vi "Check Variant Data.vi"(3 "Variant Data":variant, 5 "Dataset":T2) -> (0 "Element Type":T1, 1 "Valid Type?":bool, 2 "Number of Dimensions":i32)   [LabVIEW 2018, in "vis3d.lvlib" / "CubeLogger.lvclass"]
uses:
  CubeLogger.lvclass
  Dataset.ctl
  <vilib>/Utility/Data Type/Type Definitions/Data Type.ctl
  <vilib>/Utility/Data Type/NI_Data Type.lvlib
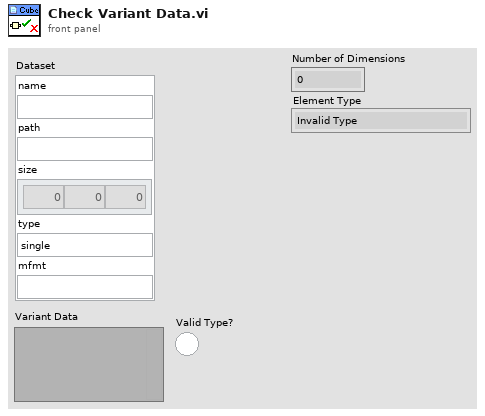
[diagram p1: front panel]
types:
  T1 = typedef "NI_Data Type.lvlib/Data Type.ctl" = enum8{"Invalid Type", "Void", "I8", "I16", "I32", "I64", "U8", "U16", "U32", "U64", "Single Float", "Double Float", "Extended Float", "Single Complex", "Double Complex", "Extended Complex", "Enum U8", "Enum U16", "Enum U32", "Enum U64", "Single Float With Unit", "Double Float With Unit", "Extended Float With Unit", "Single Complex with Unit", "Double Complex with Unit", "Extended Complex with Unit", "Boolean", "String", "Path", "Picture", "Tag", "Array", "Cluster", "Variant", "LV Variant", "Waveform", "Timestamp", "Digital Waveform", "Digital Data", "ExpressData", "Refnum", "External Data", "VI", "Poly VI", "LabVIEW Class Instance", "Fixed Point"}
  T2 = typedef "vis3d.lvlib/CubeLogger.lvclass/Dataset.ctl" = cluster{"name":string, "path":string, "size":i32[], "type":enum16{"single", "double", "uint8", "uint16", "uint32", "uint64", "int8", "int16", "int32", "int64"}, "mfmt":string}
  T3 = enum16{"single", "double", "uint8", "uint16", "uint32", "uint64", "int8", "int16", "int32", "int64"}
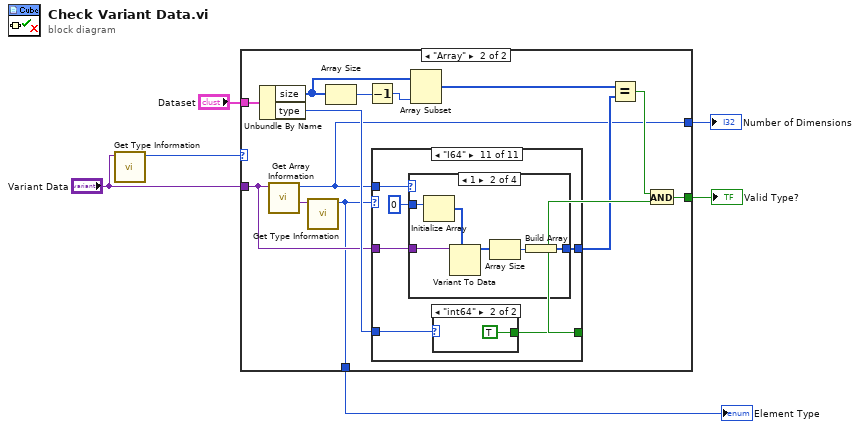
[diagram p0: block diagram]
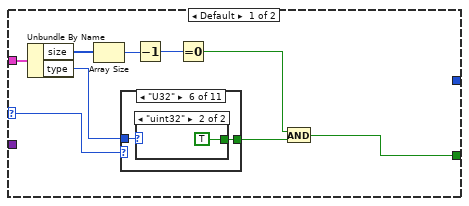
[diagram p2: hidden frame]
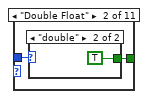
[diagram p4: hidden frame]
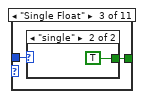
[diagram p6: hidden frame]
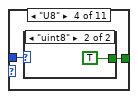
[diagram p8: hidden frame]
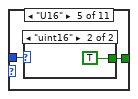
[diagram p10: hidden frame]
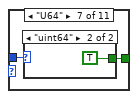
[diagram p13: hidden frame]
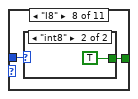
[diagram p15: hidden frame]
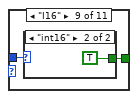
[diagram p17: hidden frame]
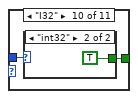
[diagram p19: hidden frame]
diagram:
  n1 = call <vilib>:"Get Type Information.vi"("Variant"="Variant Data") -> ("Type"=w6:T1)  [unwired: 6 in, 4 out]
  n2 = case shown="\"Array\"" w6 {
    selector: w6 -> [w13 _]
    tunnel: [w8 w57] -> w3
    tunnel: "Variant Data" -> [_ w49]
    tunnel: "Dataset" -> [w15 w59]
    tunnel: [_ w47] -> w2
    tunnel: [_ w46] -> w1
    frame Default {
      n3 = Unbundle By Name(w15) -> ("size"=w12:i32[], "type"=w14:T3)
      n4 = Array Size(array=w12) -> (size(s)=w11:i32)
      n5 = case shown="\"U32\"" w13 {
        tunnel: [_ w16 w19 w22 w25 w28 w31 w34 w37 w40 w43] -> w9
        tunnel: w14 -> [_ w17 w20 w23 w26 w29 w32 w35 w38 w41 w44]
        frame "Invalid Type", Default {
        }
        frame "Double Float" {
          n6 = case shown="\"double\"" w17 {
            tunnel: [_ TRUE] -> w16
            frame Default {
            }
            frame "double" {
            }
          }
        }
        frame "Single Float" {
          n7 = case shown="\"single\"" w20 {
            tunnel: [_ TRUE] -> w19
            frame Default {
            }
            frame "single" {
            }
          }
        }
        frame "U8" {
          n8 = case shown="\"uint8\"" w23 {
            tunnel: [_ TRUE] -> w22
            frame Default {
            }
            frame "uint8" {
            }
          }
        }
        frame "U16" {
          n9 = case shown="\"uint16\"" w26 {
            tunnel: [_ TRUE] -> w25
            frame Default {
            }
            frame "uint16" {
            }
          }
        }
        frame "U32" {
          n10 = case shown="\"uint32\"" w29 {
            tunnel: [_ TRUE] -> w28
            frame Default {
            }
            frame "uint32" {
            }
          }
        }
        frame "U64" {
          n11 = case shown="\"uint64\"" w32 {
            tunnel: [_ TRUE] -> w31
            frame Default {
            }
            frame "uint64" {
            }
          }
        }
        frame "I8" {
          n12 = case shown="\"int8\"" w35 {
            tunnel: [_ TRUE] -> w34
            frame Default {
            }
            frame "int8" {
            }
          }
        }
        frame "I16" {
          n13 = case shown="\"int16\"" w38 {
            tunnel: [_ TRUE] -> w37
            frame Default {
            }
            frame "int16" {
            }
          }
        }
        frame "I32" {
          n14 = case shown="\"int32\"" w41 {
            tunnel: [_ TRUE] -> w40
            frame Default {
            }
            frame "int32" {
            }
          }
        }
        frame "I64" {
          n15 = case shown="\"int64\"" w44 {
            tunnel: [_ TRUE] -> w43
            frame Default {
            }
            frame "int64" {
            }
          }
        }
      }
      n16 = Decrement(x=w11) -> (x-1=w10:i32)
      n17 = Equal To 0?(x=w10) -> (x = 0?=w7:bool)
      n18 = And(x=w7, y=w9) -> (x .and. y?=w8:bool)
    }
    frame "Array" {
      n19 = Unbundle By Name(w59) -> ("size"=w52:i32[], "type"=w54:T3)
      n20 = call <vilib>:"Get Array Information.vi"("Variant"=w49) -> ("Array Element Data Type"=w56:variant, "Number of Dimensions"=w47:i32)  [unwired: 7 in, 2 out]
      n21 = call <vilib>:"Get Type Information.vi"("Variant"=w56) -> ("Type"=w46:T1)  [unwired: 6 in, 4 out]
      n22 = Array Size(array=w52) -> (size(s)=w50:i32)
      n23 = Decrement(x=w50) -> (x-1=w51:i32)
      n24 = case shown="\"I64\"" w46 {
        tunnel: [_ w64 w87 w110 w133 w156 w179 w202 w225 w248 w271] -> w55
        tunnel: w54 -> [_ w65 w88 w111 w134 w157 w180 w203 w226 w249 w272]
        tunnel: w47 -> [_ w63 w86 w109 w132 w155 w178 w201 w224 w247 w270]
        tunnel: w49 -> [_ w61 w84 w107 w130 w153 w176 w199 w222 w245 w268]
        tunnel: [_ w60 w83 w106 w129 w152 w175 w198 w221 w244 w267] -> w48
        frame "Invalid Type", Default {
        }
        frame "Double Float" {
          n25 = case shown="1" w63 {
            tunnel: 0.0 -> [_ w69 w74 w79]
            tunnel: [_ w66 w72 w77] -> w60
            tunnel: w61 -> [_ w67 w73 w78]
            frame Default {
            }
            frame 1 {
              n26 = Initialize Array(w69) -> (w71:dbl[])  [unwired: 1 in]
              n27 = Variant To Data(type=w71, Variant=w67) -> (data=w70:dbl[])  [unwired: 1 in, 1 out]
              n28 = Array Size(array=w70) -> (size(s)=w68:i32)
              n29 = Build Array(w68) -> (w66:i32[])
            }
            frame 2 {
              n30 = Initialize Array(w74) -> (w76:dbl[][])  [unwired: 2 in]
              n31 = Variant To Data(type=w76, Variant=w73) -> (data=w75:dbl[][])  [unwired: 1 in, 1 out]
              n32 = Array Size(array=w75) -> (size(s)=w72:i32[])
            }
            frame 3 {
              n33 = Initialize Array(w79) -> (w81:dbl[][][])  [unwired: 3 in]
              n34 = Variant To Data(type=w81, Variant=w78) -> (data=w80:dbl[][][])  [unwired: 1 in, 1 out]
              n35 = Array Size(array=w80) -> (size(s)=w77:i32[])
            }
          }
          n36 = case shown="\"double\"" w65 {
            tunnel: [_ TRUE] -> w64
            frame Default {
            }
            frame "double" {
            }
          }
        }
        frame "Single Float" {
          n37 = case shown="1" w86 {
            tunnel: sgl 0.0 -> [_ w92 w97 w102]
            tunnel: [_ w89 w95 w100] -> w83
            tunnel: w84 -> [_ w90 w96 w101]
            frame Default {
            }
            frame 1 {
              n38 = Initialize Array(w92) -> (w94:sgl[])  [unwired: 1 in]
              n39 = Variant To Data(type=w94, Variant=w90) -> (data=w93:sgl[])  [unwired: 1 in, 1 out]
              n40 = Array Size(array=w93) -> (size(s)=w91:i32)
              n41 = Build Array(w91) -> (w89:i32[])
            }
            frame 2 {
              n42 = Initialize Array(w97) -> (w99:sgl[][])  [unwired: 2 in]
              n43 = Variant To Data(type=w99, Variant=w96) -> (data=w98:sgl[][])  [unwired: 1 in, 1 out]
              n44 = Array Size(array=w98) -> (size(s)=w95:i32[])
            }
            frame 3 {
              n45 = Initialize Array(w102) -> (w104:sgl[][][])  [unwired: 3 in]
              n46 = Variant To Data(type=w104, Variant=w101) -> (data=w103:sgl[][][])  [unwired: 1 in, 1 out]
              n47 = Array Size(array=w103) -> (size(s)=w100:i32[])
            }
          }
          n48 = case shown="\"single\"" w88 {
            tunnel: [_ TRUE] -> w87
            frame Default {
            }
            frame "single" {
            }
          }
        }
        frame "U8" {
          n49 = case shown="1" w109 {
            tunnel: u8 0 -> [_ w115 w120 w125]
            tunnel: [_ w112 w118 w123] -> w106
            tunnel: w107 -> [_ w113 w119 w124]
            frame Default {
            }
            frame 1 {
              n50 = Initialize Array(w115) -> (w117:u8[])  [unwired: 1 in]
              n51 = Variant To Data(type=w117, Variant=w113) -> (data=w116:u8[])  [unwired: 1 in, 1 out]
              n52 = Array Size(array=w116) -> (size(s)=w114:i32)
              n53 = Build Array(w114) -> (w112:i32[])
            }
            frame 2 {
              n54 = Initialize Array(w120) -> (w122:u8[][])  [unwired: 2 in]
              n55 = Variant To Data(type=w122, Variant=w119) -> (data=w121:u8[][])  [unwired: 1 in, 1 out]
              n56 = Array Size(array=w121) -> (size(s)=w118:i32[])
            }
            frame 3 {
              n57 = Initialize Array(w125) -> (w127:u8[][][])  [unwired: 3 in]
              n58 = Variant To Data(type=w127, Variant=w124) -> (data=w126:u8[][][])  [unwired: 1 in, 1 out]
              n59 = Array Size(array=w126) -> (size(s)=w123:i32[])
            }
          }
          n60 = case shown="\"uint8\"" w111 {
            tunnel: [_ TRUE] -> w110
            frame Default {
            }
            frame "uint8" {
            }
          }
        }
        frame "U16" {
          n61 = case shown="1" w132 {
            tunnel: u16 0 -> [_ w138 w143 w148]
            tunnel: [_ w135 w141 w146] -> w129
            tunnel: w130 -> [_ w136 w142 w147]
            frame Default {
            }
            frame 1 {
              n62 = Initialize Array(w138) -> (w140:u16[])  [unwired: 1 in]
              n63 = Variant To Data(type=w140, Variant=w136) -> (data=w139:u16[])  [unwired: 1 in, 1 out]
              n64 = Array Size(array=w139) -> (size(s)=w137:i32)
              n65 = Build Array(w137) -> (w135:i32[])
            }
            frame 2 {
              n66 = Initialize Array(w143) -> (w145:u16[][])  [unwired: 2 in]
              n67 = Variant To Data(type=w145, Variant=w142) -> (data=w144:u16[][])  [unwired: 1 in, 1 out]
              n68 = Array Size(array=w144) -> (size(s)=w141:i32[])
            }
            frame 3 {
              n69 = Initialize Array(w148) -> (w150:u16[][][])  [unwired: 3 in]
              n70 = Variant To Data(type=w150, Variant=w147) -> (data=w149:u16[][][])  [unwired: 1 in, 1 out]
              n71 = Array Size(array=w149) -> (size(s)=w146:i32[])
            }
          }
          n72 = case shown="\"uint16\"" w134 {
            tunnel: [_ TRUE] -> w133
            frame Default {
            }
            frame "uint16" {
            }
          }
        }
        frame "U32" {
          n73 = case shown="1" w155 {
            tunnel: u32 0 -> [_ w161 w166 w171]
            tunnel: [_ w158 w164 w169] -> w152
            tunnel: w153 -> [_ w159 w165 w170]
            frame Default {
            }
            frame 1 {
              n74 = Initialize Array(w161) -> (w163:u32[])  [unwired: 1 in]
              n75 = Variant To Data(type=w163, Variant=w159) -> (data=w162:u32[])  [unwired: 1 in, 1 out]
              n76 = Array Size(array=w162) -> (size(s)=w160:i32)
              n77 = Build Array(w160) -> (w158:i32[])
            }
            frame 2 {
              n78 = Initialize Array(w166) -> (w168:u32[][])  [unwired: 2 in]
              n79 = Variant To Data(type=w168, Variant=w165) -> (data=w167:u32[][])  [unwired: 1 in, 1 out]
              n80 = Array Size(array=w167) -> (size(s)=w164:i32[])
            }
            frame 3 {
              n81 = Initialize Array(w171) -> (w173:u32[][][])  [unwired: 3 in]
              n82 = Variant To Data(type=w173, Variant=w170) -> (data=w172:u32[][][])  [unwired: 1 in, 1 out]
              n83 = Array Size(array=w172) -> (size(s)=w169:i32[])
            }
          }
          n84 = case shown="\"uint32\"" w157 {
            tunnel: [_ TRUE] -> w156
            frame Default {
            }
            frame "uint32" {
            }
          }
        }
        frame "U64" {
          n85 = case shown="1" w178 {
            tunnel: u64 0 -> [_ w184 w189 w194]
            tunnel: [_ w181 w187 w192] -> w175
            tunnel: w176 -> [_ w182 w188 w193]
            frame Default {
            }
            frame 1 {
              n86 = Initialize Array(w184) -> (w186:u64[])  [unwired: 1 in]
              n87 = Variant To Data(type=w186, Variant=w182) -> (data=w185:u64[])  [unwired: 1 in, 1 out]
              n88 = Array Size(array=w185) -> (size(s)=w183:i32)
              n89 = Build Array(w183) -> (w181:i32[])
            }
            frame 2 {
              n90 = Initialize Array(w189) -> (w191:u64[][])  [unwired: 2 in]
              n91 = Variant To Data(type=w191, Variant=w188) -> (data=w190:u64[][])  [unwired: 1 in, 1 out]
              n92 = Array Size(array=w190) -> (size(s)=w187:i32[])
            }
            frame 3 {
              n93 = Initialize Array(w194) -> (w196:u64[][][])  [unwired: 3 in]
              n94 = Variant To Data(type=w196, Variant=w193) -> (data=w195:u64[][][])  [unwired: 1 in, 1 out]
              n95 = Array Size(array=w195) -> (size(s)=w192:i32[])
            }
          }
          n96 = case shown="\"uint64\"" w180 {
            tunnel: [_ TRUE] -> w179
            frame Default {
            }
            frame "uint64" {
            }
          }
        }
        frame "I8" {
          n97 = case shown="1" w201 {
            tunnel: i8 0 -> [_ w207 w212 w217]
            tunnel: [_ w204 w210 w215] -> w198
            tunnel: w199 -> [_ w205 w211 w216]
            frame Default {
            }
            frame 1 {
              n98 = Initialize Array(w207) -> (w209:i8[])  [unwired: 1 in]
              n99 = Variant To Data(type=w209, Variant=w205) -> (data=w208:i8[])  [unwired: 1 in, 1 out]
              n100 = Array Size(array=w208) -> (size(s)=w206:i32)
              n101 = Build Array(w206) -> (w204:i32[])
            }
            frame 2 {
              n102 = Initialize Array(w212) -> (w214:i8[][])  [unwired: 2 in]
              n103 = Variant To Data(type=w214, Variant=w211) -> (data=w213:i8[][])  [unwired: 1 in, 1 out]
              n104 = Array Size(array=w213) -> (size(s)=w210:i32[])
            }
            frame 3 {
              n105 = Initialize Array(w217) -> (w219:i8[][][])  [unwired: 3 in]
              n106 = Variant To Data(type=w219, Variant=w216) -> (data=w218:i8[][][])  [unwired: 1 in, 1 out]
              n107 = Array Size(array=w218) -> (size(s)=w215:i32[])
            }
          }
          n108 = case shown="\"int8\"" w203 {
            tunnel: [_ TRUE] -> w202
            frame Default {
            }
            frame "int8" {
            }
          }
        }
        frame "I16" {
          n109 = case shown="1" w224 {
            tunnel: i16 0 -> [_ w230 w235 w240]
            tunnel: [_ w227 w233 w238] -> w221
            tunnel: w222 -> [_ w228 w234 w239]
            frame Default {
            }
            frame 1 {
              n110 = Initialize Array(w230) -> (w232:i16[])  [unwired: 1 in]
              n111 = Variant To Data(type=w232, Variant=w228) -> (data=w231:i16[])  [unwired: 1 in, 1 out]
              n112 = Array Size(array=w231) -> (size(s)=w229:i32)
              n113 = Build Array(w229) -> (w227:i32[])
            }
            frame 2 {
              n114 = Initialize Array(w235) -> (w237:i16[][])  [unwired: 2 in]
              n115 = Variant To Data(type=w237, Variant=w234) -> (data=w236:i16[][])  [unwired: 1 in, 1 out]
              n116 = Array Size(array=w236) -> (size(s)=w233:i32[])
            }
            frame 3 {
              n117 = Initialize Array(w240) -> (w242:i16[][][])  [unwired: 3 in]
              n118 = Variant To Data(type=w242, Variant=w239) -> (data=w241:i16[][][])  [unwired: 1 in, 1 out]
              n119 = Array Size(array=w241) -> (size(s)=w238:i32[])
            }
          }
          n120 = case shown="\"int16\"" w226 {
            tunnel: [_ TRUE] -> w225
            frame Default {
            }
            frame "int16" {
            }
          }
        }
        frame "I32" {
          n121 = case shown="1" w247 {
            tunnel: 0 -> [_ w253 w258 w263]
            tunnel: [_ w250 w256 w261] -> w244
            tunnel: w245 -> [_ w251 w257 w262]
            frame Default {
            }
            frame 1 {
              n122 = Initialize Array(w253) -> (w255:i32[])  [unwired: 1 in]
              n123 = Variant To Data(type=w255, Variant=w251) -> (data=w254:i32[])  [unwired: 1 in, 1 out]
              n124 = Array Size(array=w254) -> (size(s)=w252:i32)
              n125 = Build Array(w252) -> (w250:i32[])
            }
            frame 2 {
              n126 = Initialize Array(w258) -> (w260:i32[][])  [unwired: 2 in]
              n127 = Variant To Data(type=w260, Variant=w257) -> (data=w259:i32[][])  [unwired: 1 in, 1 out]
              n128 = Array Size(array=w259) -> (size(s)=w256:i32[])
            }
            frame 3 {
              n129 = Initialize Array(w263) -> (w265:i32[][][])  [unwired: 3 in]
              n130 = Variant To Data(type=w265, Variant=w262) -> (data=w264:i32[][][])  [unwired: 1 in, 1 out]
              n131 = Array Size(array=w264) -> (size(s)=w261:i32[])
            }
          }
          n132 = case shown="\"int32\"" w249 {
            tunnel: [_ TRUE] -> w248
            frame Default {
            }
            frame "int32" {
            }
          }
        }
        frame "I64" {
          n133 = case shown="1" w270 {
            tunnel: i64 0 -> [_ w276 w281 w286]
            tunnel: [_ w273 w279 w284] -> w267
            tunnel: w268 -> [_ w274 w280 w285]
            frame Default {
            }
            frame 1 {
              n134 = Initialize Array(w276) -> (w278:i64[])  [unwired: 1 in]
              n135 = Variant To Data(type=w278, Variant=w274) -> (data=w277:i64[])  [unwired: 1 in, 1 out]
              n136 = Array Size(array=w277) -> (size(s)=w275:i32)
              n137 = Build Array(w275) -> (w273:i32[])
            }
            frame 2 {
              n138 = Initialize Array(w281) -> (w283:i64[][])  [unwired: 2 in]
              n139 = Variant To Data(type=w283, Variant=w280) -> (data=w282:i64[][])  [unwired: 1 in, 1 out]
              n140 = Array Size(array=w282) -> (size(s)=w279:i32[])
            }
            frame 3 {
              n141 = Initialize Array(w286) -> (w288:i64[][][])  [unwired: 3 in]
              n142 = Variant To Data(type=w288, Variant=w285) -> (data=w287:i64[][][])  [unwired: 1 in, 1 out]
              n143 = Array Size(array=w287) -> (size(s)=w284:i32[])
            }
          }
          n144 = case shown="\"int64\"" w272 {
            tunnel: [_ TRUE] -> w271
            frame Default {
            }
            frame "int64" {
            }
          }
        }
      }
      n145 = Array Subset(array=w52, length=w51) -> (w53:i32[])  [unwired: 1 in]
      n146 = Equal?(x=w53, y=w48) -> (x = y?=w58:bool)
      n147 = And(x=w58, y=w55) -> (x .and. y?=w57:bool)
    }
  }
  "Valid Type?" <- w3
  "Number of Dimensions" <- w2
  "Element Type" <- w1
